vi "All Cluster Groups.vi"(8 "error in (no error)":errorcluster, 9 "Cluster Name":string, 11 "VolatusConfig in":refnum<class "VolatusConfig.lvclass">) -> (0 "error out":errorcluster, 2 "Groups":refnum<class "Group Config.lvclass">[](array[class]), 3 "VolatusConfig out":refnum<class "VolatusConfig.lvclass">)   [LabVIEW 2023, in "VolatusConfig.lvlib" / "VolatusConfig.lvclass"]
uses:
  VolatusConfig.lvclass
  Group/Group Config.lvclass
  Meta Type.ctl
  VolatusConfig.lvclass/VolatusConfig.ctl
  lv-cdm/CDM-Config/Config Lookup/Match Meta.vi
  lv-cdm/CDM-Config/Config Manager/Lookup Descendant.vi
  lv-cdm/CDM-Config/Config Filter/Config Lookup.lvclass
  VolatusConfig.lvlib
  lv-cdm/CDM-Config/Config Element/Config Element.lvclass
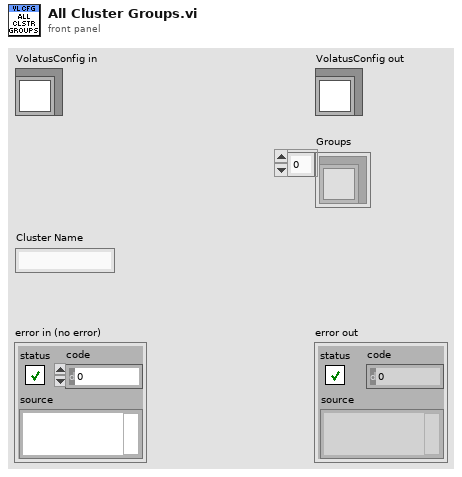
[diagram p1: front panel]
types:
  T1 = typedef "VolatusConfig.lvlib/Meta Type.ctl" = enum16{"UNKNOWN", "VL_System", "VL_Cluster", "VL_Node", "VL_Task", "VL_Group", "VL_Channel", "VL_Task_List", "VL_Scaling", "VL_Sensor", "VL_Sensor_List", "VL_Scale"}
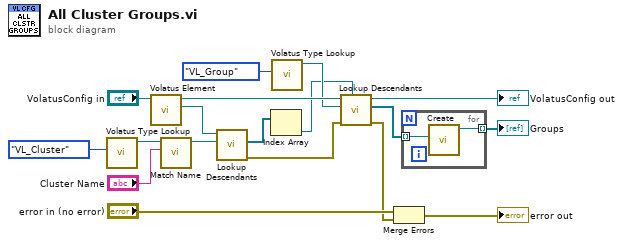
[diagram p0: block diagram]
diagram:
  n1 = call "Volatus Type Lookup.vi"("Meta Type"=Meta_Type."VL_Cluster") -> ("Config Lookup out"=w6:refnum<class "Config Lookup.lvclass">)  [unwired: 9 in, 1 out]
  n2 = call "Volatus Element.vi"("VolatusConfig in"="VolatusConfig in") -> ("Volatus Element"=w7:refnum<class "Config Element.lvclass">, "VolatusConfig out"=w16:refnum<class "VolatusConfig.lvclass">)  [unwired: 8 in, 1 out]
  n3 = call "Match Name.vi"("Name"="Cluster Name", "Config Lookup (New)"=w6) -> ("Config Lookup out"=w4:refnum<class "Config Lookup.lvclass">)  [unwired: 8 in, 1 out]
  n4 = call "Lookup Descendants.vi"("Lookup"=w4, "Config Element in"=w7) -> ("error out"=w3:errorcluster, "Descendants"=w2:refnum<class "Config Element.lvclass">[])  [unwired: 7 in, 1 out]
  n5 = Index Array(array=w2) -> (element=w1:refnum<class "Config Element.lvclass">)  [unwired: 1 in]
  n6 = call "Volatus Type Lookup.vi"("Meta Type"=Meta_Type."VL_Group") -> ("Config Lookup out"=w13:refnum<class "Config Lookup.lvclass">)  [unwired: 9 in, 1 out]
  n7 = call "Lookup Descendants.vi"("Start (Root)"=w1, "error in (no error)"=w3, "Lookup"=w13, "VolatusConfig in"=w16) -> ("error out"=w9:errorcluster, "Descendants"=w12:refnum<class "Config Element.lvclass">[], "VolatusConfig out"=→"VolatusConfig out":refnum<class "VolatusConfig.lvclass">)  [unwired: 5 in]
  n8 = Merge Errors("error in (no error)", w9) -> (→"error out":errorcluster)
  n9 = for {
    tunnel: w12 -> [w20] mode=indexing
    tunnel: [w19] -> w11 mode=indexing
    n10 = call "Create.vi"("Element"=w20) -> ("Group out"=w19:refnum<class "Group Config.lvclass">)  [unwired: 9 in, 1 out]
  }
  "Groups" <- w11
